vi "Server Parse Commands.vi"(8 "error in":errorcluster, 11 "string":string) -> (0 "error out":errorcluster, 1 "command string":string, 2 "command data":string, 3 "command":T1=enum."Reset")   [LabVIEW 2013]
doc: "Parse server command. It will detect command ID and extract its data."
uses:
  Server Event Command.ctl
  <vilib>/Utility/error.llb/Error Cluster From Error Code.vi
  <vilib>/regexp/Match Regular Expression.xnode
  <vilib>/ErrorRing/Error Ring.xnode
  octave/infolib.lvlibp
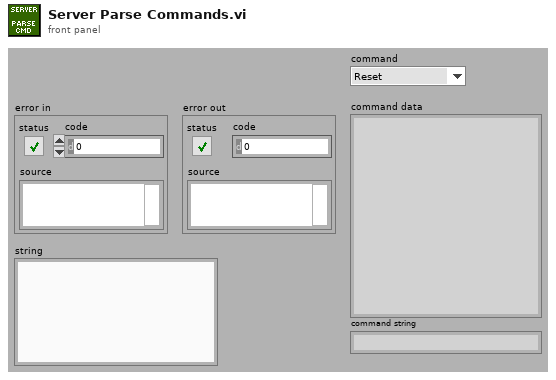
[diagram p1: front panel]
types:
  T1 = typedef "Server Event Command.ctl" = enum16{"None", "Reset", "Identify", "Start", "Get status", "Get result"}
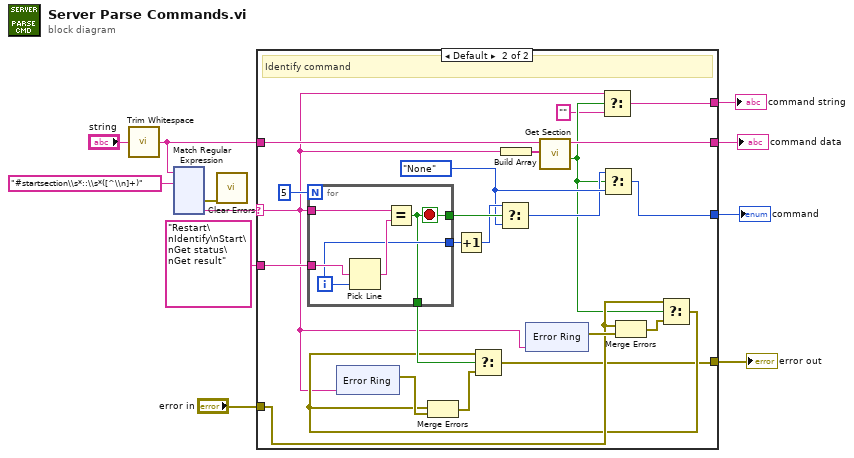
[diagram p0: block diagram]
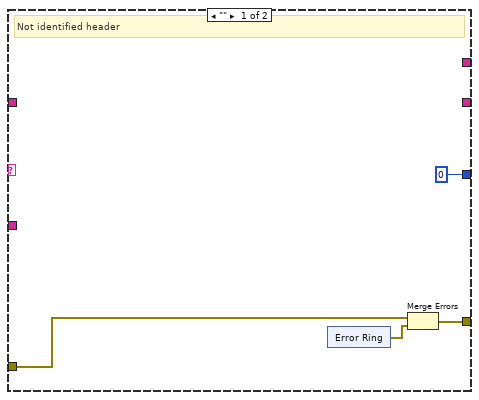
[diagram p2: hidden frame]
diagram:
  n1 = call <vilib>:"Trim Whitespace.vi"("string"="string") -> ("trimmed string"=w5:string)  [unwired: 1 in]
  n2 = xnode "Match Regular Expression"("input string"=w5, "regular expression"="#startsection\\s*::\\s*([^\\n]+)") -> ("error out"=w1:errorcluster, "submatch 1"=w8:string)  [unwired: 4 in, 4 out]
  n3 = call <vilib>:"Clear Errors.vi"("error in (no error)"=w1) -> ()  [unwired: 6 in, 1 out]
  n4 = case shown="Default" w8 {
    selector: w8 -> [_ w22]
    tunnel: "Restart\nIdentify\nStart\nGet status\nGet result" -> [_ w43]
    tunnel: "error in" -> [w13 w27]
    tunnel: [0 w30] -> w6
    tunnel: w5 -> [_ w36]
    tunnel: [_ w34] -> w4
    tunnel: [w14 w25] -> w3
    tunnel: [_ w24] -> w2
    frame "" {
      # "Not identified header"
      n5 = xnode "Error Ring"() -> ("error out"=w12:errorcluster)
      n6 = Merge Errors(w13, w12) -> (w14:errorcluster)
    }
    frame Default {
      w32 = Server_Event_Command."None" ("command")
      # "Identify command"
      n7 = for {
        N: 5 -> [_]
        tunnel: w43 -> [w62]
        tunnel: w22 -> [w60]
        tunnel: [w59] -> w42
        tunnel: [w58] -> w41
        tunnel: [w58] -> w38
        i -> [w59]
        stop <- w58 stop-if-true
        n8 = Pick Line(multi-line string=w62, line index=w59) -> (output string=w61:string)  [unwired: 1 in]
        n9 = Equal?(x=w60, y=w61) -> (x = y?=w58:bool)
      }
      n10 = xnode "Error Ring"("parameter 0"=w22) -> ("error out"=w40:errorcluster)
      n11 = Increment(x=w42) -> (x+1=w37:i32)
      n12 = Select(t=w37, s=w38, f=w32) -> (s? t:f=w31:i32)
      n13 = Build Array(w22) -> (w35:string[])
      n14 = xnode "Error Ring"("parameter 0"=w22) -> ("error out"=w28:errorcluster)
      n15 = call "Get Section.vi"("sections"=w35, "info data"=w36) -> ("exist"=w23:bool, "section part"=w34:string)  [unwired: 8 in]
      n16 = Select(t=w22, s=w23, f="") -> (s? t:f=w24:string)
      n17 = Select(t=w31, s=w23, f=w32) -> (s? t:f=w30:i32)
      n18 = Merge Errors(w27, w28) -> (w29:errorcluster)
      n19 = Select(t=w27, s=w23, f=w29) -> (s? t:f=w26:errorcluster)
      n20 = Merge Errors(w26, w40) -> (w39:errorcluster)
      n21 = Select(t=w26, s=w41, f=w39) -> (s? t:f=w25:errorcluster)
    }
  }
  "error out" <- w3
  "command" <- w6
  "command data" <- w4
  "command string" <- w2
